vi "WinCI Close Project.vi"(8 "error in (no error)":errorcluster, 11 "source control reference in":T1) -> (0 "error out":errorcluster, 2 "status message":string)   [LabVIEW 2020, in "NI_SCC_WinCI.lvlib"]
uses:
  <vilib>/SourceControl/Providers/WinCI/NI_SCC_WinCI.lvlib
  <vilib>/SourceControl/sccapi/SCCAPI Refnum.ctl
  <vilib>/SourceControl/support/SCCSup Message Strings GLBL.vi
  <vilib>/SourceControl/sccapi/NI_SCC.lvlib
panel:
  out "result":i32
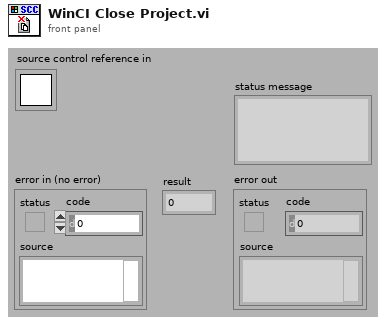
[diagram p1: front panel]
types:
  T1 = typedef "NI_SCC.lvlib/SCCAPI Refnum.ctl" = refnum<k1>
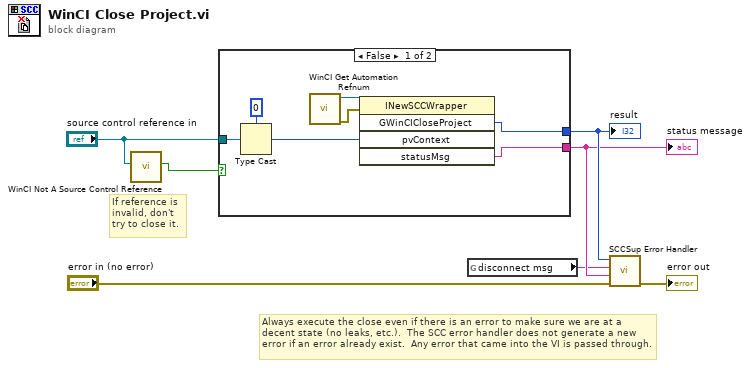
[diagram p0: block diagram]
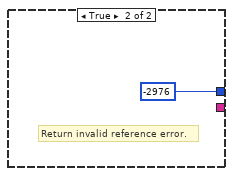
[diagram p2: hidden frame]
diagram:
  # "If reference is invalid, don't try to close it."
  # "Always execute the close even if there is an error to make sure we are at a decent state (no leaks, etc.).  The SCC error handler does not generate a new error if an error already exist.  Any error that came into the VI is passed through."
  n1 = call <vilib>:"WinCI Not A Source Control Reference.vi"("source control reference in"="source control reference in") -> ("not a source control reference?"=w1:bool)  [unwired: 1 in, 9 out]
  n2 = case shown="False" w1 {
    tunnel: [w11 -2976 ("result")] -> w7
    tunnel: [w10 _] -> w5
    tunnel: "source control reference in" -> [w13 _]
    frame False {
      n3 = Type Cast(type=u32 0, x=w13) -> (*(type *) &x=w12:u32)
      n4 = call <vilib>:"WinCI Get Automation Refnum.vi"() -> ("error out"=w9:errorcluster, "automation refnum"=w8:refnum<k7>)  [unwired: 10 out]
      n5 = invoke class="INewSCCWrapper" method="GWinCICloseProject"(reference=w8, error in=w9, "pvContext"=w12) -> ("GWinCICloseProject"=w11:i32, "statusMsg"=w10:string)  [unwired: 2 in, 3 out]
    }
    frame True {
      # "Return invalid reference error."
    }
  }
  "status message" <- w5
  "result" <- w7
  n6 = global read "SCCSup Message Strings GLBL.vi" "disconnect msg"() -> (w4:string)
  n7 = call <vilib>:"SCCSup Error Handler.vi"("error in (no error)"="error in (no error)", "additional message"=w5, "operation message"=w4, "scc error code"=w7) -> ("error out"=→"error out":errorcluster)  [unwired: 7 out]
